vi "picoscope5000a acquire.vi"(0 "handle in":i16, 1 "Ranges":u16[](array[numeric])=[6, 6], 5 "enabled array":i16[](array[numeric]), 7 "Max ADC value":i16, 9 "Device Info":T2, 11 "error in (no error)":errorcluster, 12 "Rapid Block Acquisition Settings":T1) -> (4 "Properties Panel":T3, 6 "handle out 2":i16, 8 "Waveform Data":waveform(dbl)[](graph), 10 "Number of Samples \nPer Capture":u32, 15 "error out":errorcluster)   [LabVIEW 2020]
panel:
  out "Rapid Block Acquisition Settings 2":T1={"preTriggerSamples"=0, "postTriggerSamples"=1000, "timebase"=2, "Down-Sample Mode"=0, "Down Sample Ratio"=1, "Number of Captures"=10} {"Down Sample Ratio" min=1 step=1; "Down-Sample Mode" items=["None"=0, "Aggregate"=1, "Decimate"=2, "Average"=4]}
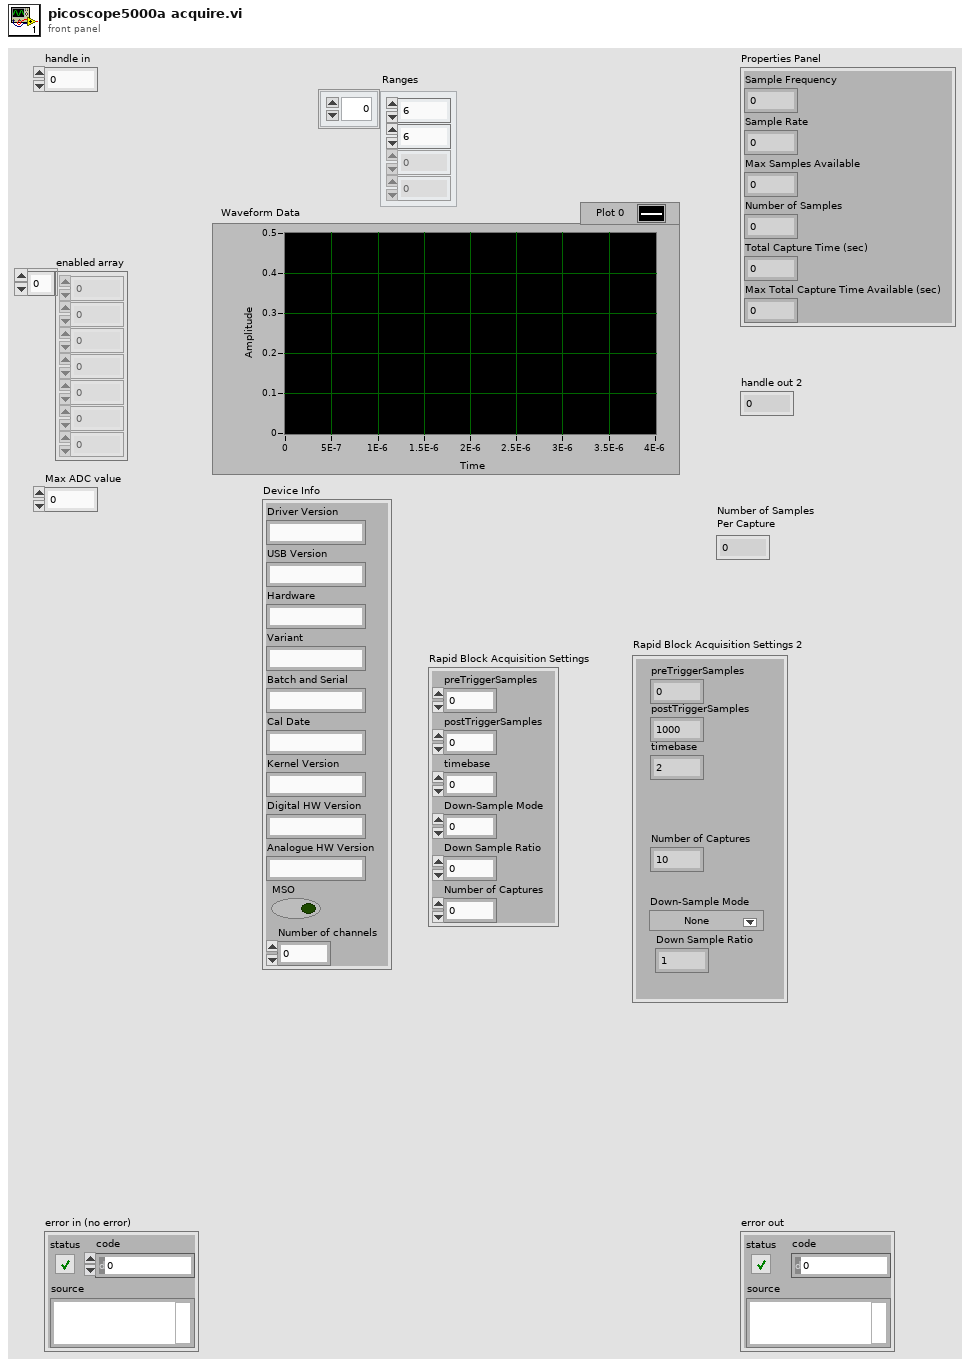
[diagram p1: front panel]
types:
  T1 = cluster{"preTriggerSamples":u32, "postTriggerSamples":u32, "timebase":u32, "Down-Sample Mode":i32, "Down Sample Ratio":u32, "Number of Captures":u32}
  T2 = cluster{"Driver Version":string, "USB Version":string, "Hardware":string, "Variant":string, "Batch and Serial":string, "Cal Date":string, "Kernel Version":string, "Digital HW Version":string, "Analogue HW Version":string, "MSO":bool, "Number of channels":i16}
  T3 = cluster{"Sample Frequency":sgl, "Sample Rate":sgl, "Max Samples Available":i32, "Number of Samples":u32, "Total Capture Time (sec) ":sgl, "Max Total Capture Time Available (sec)":sgl}
  T4 = cluster{"preTriggerSamples":u32, "postTriggerSamples":u32, "timebase":u32, "Down-Sample Mode":i32, "Down Sample Ratio":u32}
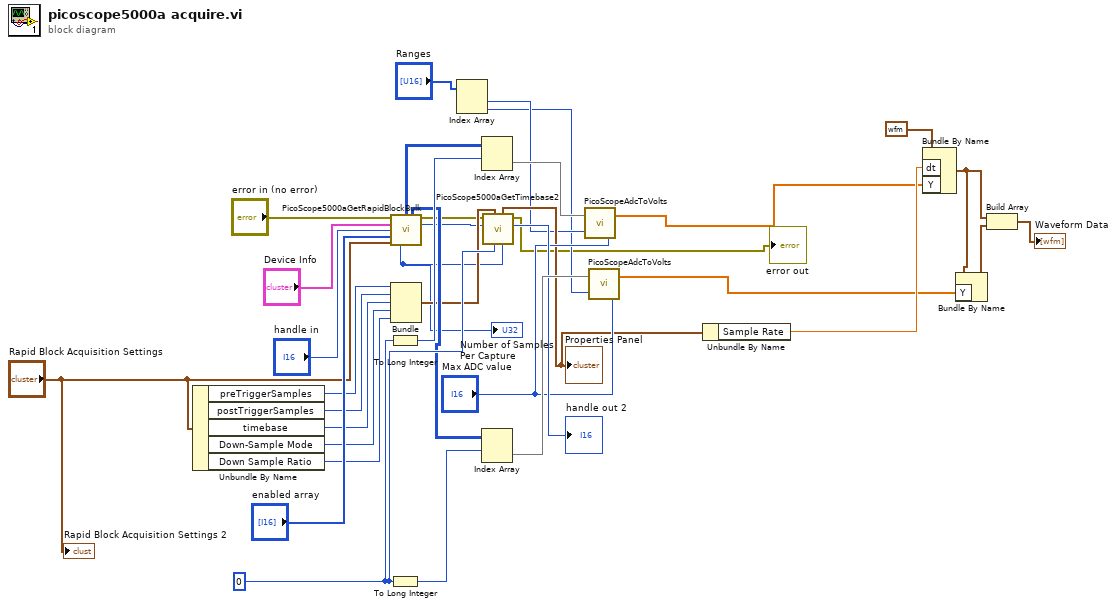
[diagram p0: block diagram]
diagram:
  w35 = i16 0 ("Capture Index")
  n1 = Unbundle By Name("Rapid Block Acquisition Settings") -> ("preTriggerSamples"=w24:u32, "postTriggerSamples"=w25:u32, "timebase"=w26:u32, "Down-Sample Mode"=w27:i32, "Down Sample Ratio"=w28:u32)
  n2 = To Long Integer(number=w35) -> (32bit integer=w32:i32)
  n3 = To Long Integer(number=w35) -> (32bit integer=w33:i32)
  n4 = call "PicoScope5000aGetRapidBlockBulk.vi"("error in"="error in (no error)", "Device Info"="Device Info", "handle in"="handle in", "enabled array"="enabled array", "Rapid Block Acquisition Settings"="Rapid Block Acquisition Settings") -> ("Channel A Buffer"=w15:i16[][], "Channel B Buffer"=w30:i16[][], "error out"=w14:errorcluster, "handle out"=w20:i16, "Num samples"=w19:u32)  [unwired: 2 in, 4 out]
  "Number of Samples \nPer Capture" <- w19
  n5 = Bundle("preTriggerSamples"=w24, "postTriggerSamples"=w25, "timebase"=w26, "Down-Sample Mode"=w27, "Down Sample Ratio"=w28) -> (w23:T4)  [unwired: 1 in]
  n6 = Index Array(array="Ranges") -> (element #1=w4:u16, element #2=w3:u16)  [unwired: 2 in]
  n7 = Index Array(array=w15, index (row)=w32) -> (element=w31:i16[])  [unwired: 1 in]
  n8 = Index Array(array=w30, index (row)=w33) -> (element=w34:i16[])  [unwired: 1 in]
  n9 = call "PicoScope5000aGetTimebase2.vi"("Number of Samples"=w19, "Memory Segment"=w35, "Acquisition Settings"=w23, "handle in"=w20, "error in (no error)"=w14) -> ("handle out"=→"handle out 2":i16, "error out"=→"error out":errorcluster, "Properties Panel"=w12:T3)  [unwired: 4 in]
  "Properties Panel" <- w12
  n10 = call "PicoScopeAdcToVolts.vi"("Max_adc"="Max ADC value", "Range Index"=w4, "Data"=w31) -> ("Data (Volts)"=w10:dbl[])
  n11 = call "PicoScopeAdcToVolts.vi"("Max_adc"="Max ADC value", "Range Index"=w3, "Data"=w34) -> ("Data (Volts)"=w8:dbl[])
  n12 = Unbundle By Name(w12) -> ("Sample Rate"=w11:sgl)
  n13 = Bundle By Name(cluster=waveform(dbl) {"t0"=timestamp(0 s since 1904-01-01), "dt"=1.0, "Y"=[]} ("Waveform Graph"), "dt"=w11, "Y"=w10) -> (w7:waveform(dbl))
  n14 = Bundle By Name(cluster=w7, "Y"=w8) -> (w6:waveform(dbl))
  n15 = Build Array(w7, w6) -> (→"Waveform Data":waveform(dbl)[])
  "Rapid Block Acquisition Settings 2" <- "Rapid Block Acquisition Settings"
